vi "AgingStatus.vi"() -> ()   [LabVIEW 2020]
panel:
  in  "StatusVJV":dbl[][](array[numeric])
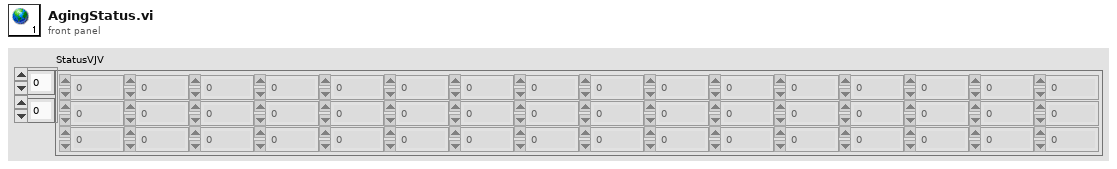
[diagram p1: front panel]
diagram:
